vi "枚举控件字号自适应.vi"(6 "留白（7）":i16=7, 7 "新旧尺寸信息":T1, 8 "错误输入（无错误）":errorcluster, 11 "枚举控件-引用":refnum<vi>) -> (0 "错误输出":errorcluster, 3 "字号":u32)   [LabVIEW 2017]
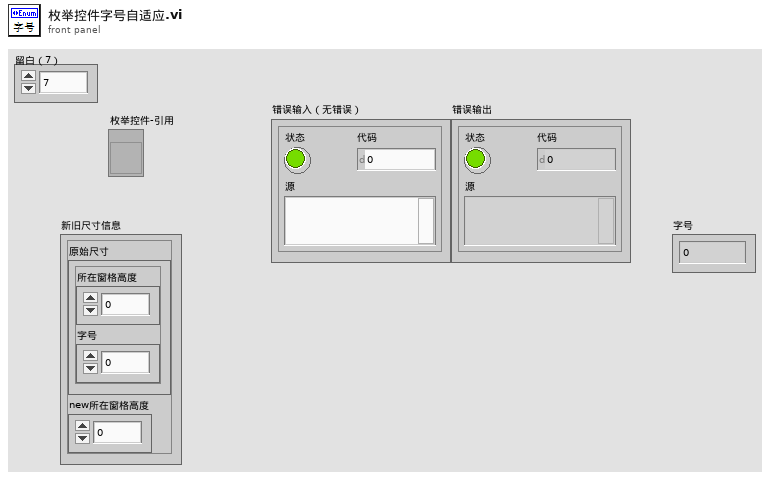
[diagram p1: front panel]
types:
  T1 = cluster{"原始尺寸":cluster{"所在窗格高度":u32, "字号":u32}, "new所在窗格高度":u32}
  T2 = typedef "LVRectTypeDef.ctl" = cluster{"Left":i16, "Top":i16, "Right":i16, "Bottom":i16}
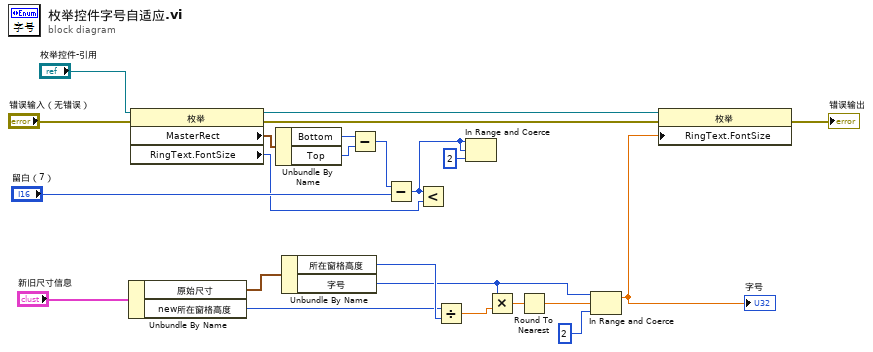
[diagram p0: block diagram]
diagram:
  n1 = Unbundle By Name("新旧尺寸信息") -> ("原始尺寸"=w6:cluster{"所在窗格高度":u32, "字号":u32}, "new所在窗格高度"=w7:u32)
  n2 = property class="枚举"(reference="枚举控件-引用", error in="错误输入（无错误）") -> (reference out=w17:refnum<vi>, error out=w16:errorcluster, "MasterRect"=w18:T2, "RingText.FontSize"=w13:u32)
  n3 = Unbundle By Name(w18) -> ("Bottom"=w21:i16, "Top"=w22:i16)
  n4 = Unbundle By Name(w6) -> ("所在窗格高度"=w8:u32, "字号"=w3:u32)
  n5 = Subtract(x=w21, y=w22) -> (x-y=w20:i16)
  n6 = Subtract(x=w20, y="留白（7）") -> (x-y=w11:i16)
  n7 = Less?(x=w11, y=w13) -> ()  [unwired: 1 out]
  n8 = Divide(x=w7, y=w8) -> (x/y=w9:dbl)
  n9 = In Range and Coerce(upper limit=w11, x=w11, lower limit=i16 2 ("下限")) -> ()  [unwired: 2 out]
  n10 = Multiply(x=w3, y=w9) -> (x*y=w10:dbl)
  n11 = Round To Nearest(number=w10) -> (nearest integer value=w2:dbl)
  n12 = In Range and Coerce(upper limit=w3, x=w2, lower limit=i16 2 ("下限")) -> (coerced(x)=w1:dbl)  [unwired: 1 out]
  "字号" <- w1
  n13 = property class="枚举"(reference=w17, error in=w16, "RingText.FontSize"=w1) -> (error out=→"错误输出":errorcluster)  [unwired: 1 out]
